vi "Vertical Insert 2.vi"(4 "Side":T1=enum."right", 7 "MaxAngle":dbl=40.0, 8 "error in":errorcluster, 9 "Speed":dbl=10.0, 10 "depth":dbl, 11 "deg/mm":dbl=10.0) -> (0 "error out":errorcluster)   [LabVIEW 2013]
uses:
  ROS/Code/SubVIs/BaxterSide.ctl
  ROS/Code/Console/Servers/ServerSubs/(nist) Arm Globals.vi
  Prim/Fwd Kenimatics - array.vi
  <vilib>/Analysis/Matrix/Numeric/Multiply/Multiply - RM,RM.vi
  Move Matrix.vi
  <vilib>/Analysis/Matrix/NI_Matrix.lvlib
panel:
  out "N":i32
  out "Array":string[](array[string])
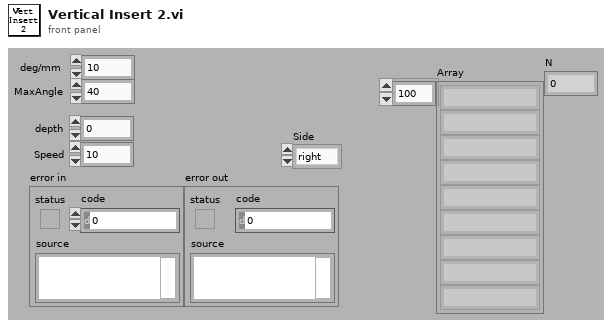
[diagram p1: front panel]
types:
  T1 = typedef "BaxterSide.ctl" = enum16{"left", "right"}
  T2 = typedef "NI_Matrix.lvlib/RealMatrix.ctl" = dbl[][]
  T3 = cluster{"X":dbl, "Y":dbl, "Z":dbl, "Roll":dbl, "Pitch":dbl, "Yaw":dbl}
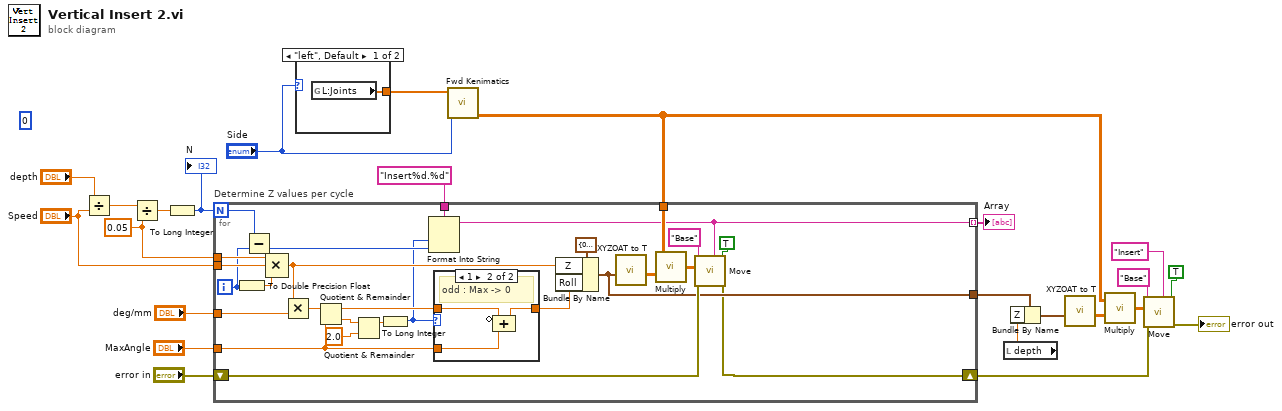
[diagram p0: block diagram]
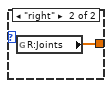
[diagram p3: hidden frame]
diagram:
  w18 = 0.05 ("y")
  (unwired) 0
  n1 = Divide(x="depth", y="Speed") -> (x/y=w21:dbl)
  n2 = Divide(x=w21, y=w18) -> (x/y=w20:dbl)
  n3 = To Long Integer(number=w20) -> (32bit integer=w19:i32)
  "N" <- w19
  n4 = case shown="\"left\", Default" "Side" {
    tunnel: [w25 w26] -> w24
    frame "left", Default {
      n5 = global read "(nist) Arm Globals.vi" "L:Joints"() -> (w25:dbl[])
    }
    frame "right" {
      n6 = global read "(nist) Arm Globals.vi" "R:Joints"() -> (w26:dbl[])
    }
  }
  n7 = call-poly "Fwd Kenimatics.vi"("Side"="Side", "Joints"=w24) -> ("Matrix"=w4:T2)  [unwired: 8 in, 1 out]
  n8 = for "Determine Z values per cycle" {
    N: w19 -> [w34]
    tunnel: w18 -> [w52]
    tunnel: "Speed" -> [w51]
    tunnel: "deg/mm" -> [w50]
    tunnel: "MaxAngle" -> [w44]
    shift-right: [w27] -> w6
    shift-left: "error in" -> [w36]
    tunnel: w4 -> [w37]
    tunnel: "Insert%d.%d" ("format string") -> [w35]
    tunnel: [w29] -> w3
    tunnel: [w30] -> w1 mode=indexing
    i -> [w33]
    n9 = To Double Precision Float(number=w33) -> (double precision float=w53:dbl)
    n10 = Subtract(x=w34, y=w33) -> (x-y=w32:i32)
    n11 = Compound Arithmetic op=MULTIPLY(w52, w51, w53) -> (w42:dbl)
    n12 = Multiply(x=w42, y=w50) -> (x*y=w49:dbl)
    n13 = Quotient & Remainder(x=w49, y=w44) -> (x-y*floor(x/y)=w45:dbl, floor(x/y)=w48:dbl)
    n14 = Quotient & Remainder(x=w48, y=2.0) -> (x-y*floor(x/y)=w46:dbl)  [unwired: 1 out]
    n15 = To Long Integer(number=w46) -> (32bit integer=w31:i32)
    n16 = Format Into String(format string=w35, w31, w32) -> (resulting string=w30:string)  [unwired: 2 in, 1 out]
    n17 = case shown="1" w31 {
      tunnel: w45 -> [w54 w57]
      tunnel: [w54 w56] -> w43
      tunnel: w44 -> [_ w55]
      frame Default {
        # "even : 0->Max"
      }
      frame 1 {
        # "odd : Max -> 0"
        n18 = Compound Arithmetic op=ADD(invert w57, w55) -> (w56:dbl)
      }
    }
    n19 = Bundle By Name(cluster=T3 {"X"=0.0, "Y"=0.0, "Z"=0.0, "Roll"=0.0, "Pitch"=0.0, "Yaw"=0.0} ("XYZOAT"), "Z"=w42, "Roll"=w43) -> (w29:T3)
    n20 = call "XYZOAT to T.vi"("XYZOAT"=w29) -> ("T"=w38:T2)  [unwired: 10 in]
    n21 = call-poly <vilib>:"Multiply.vi"("Real Matrix B"=w38, "Real Matrix A"=w37) -> ("A * B"=w39:T2)
    n22 = call-poly "Move.vi"("Make Vertical"=TRUE, "Label"=w30, "error in"=w36, "Offset"=w39, "Location"="Base") -> ("error out"=w27:errorcluster)  [unwired: 6 in]
  }
  "Array" <- w1
  n23 = local read "depth"() -> (w2:dbl)
  n24 = Bundle By Name(cluster=w3, "Z"=w2) -> (w12:T3)
  n25 = call "XYZOAT to T.vi"("XYZOAT"=w12) -> ("T"=w8:T2)  [unwired: 10 in]
  n26 = call-poly <vilib>:"Multiply.vi"("Real Matrix B"=w8, "Real Matrix A"=w4) -> ("A * B"=w10:T2)
  n27 = call-poly "Move.vi"("Make Vertical"=TRUE, "Label"="Insert", "error in"=w6, "Offset"=w10, "Location"="Base") -> ("error out"=→"error out":errorcluster)  [unwired: 6 in]
